vi "Calculate Values Of ScrollBar.vi"(9 "Bounds  Of Picture":T1, 10 "Display Data":T2[](array[typedef]), 11 "Actual Data":T2[](array[typedef])) -> (2 "Total":u32, 3 "index of element":i32, 4 "Max.Scale":i32)   [LabVIEW 2014, in "SmartPalette.lvlib"]
uses:
  SmartPalette.lvlib
  Controls/Palette Data.ctl
  <vilib>/picture/picture.llb/imagedata.ctl
  <vilib>/Utility/miscctls.llb/LVBoundsTypeDef.ctl
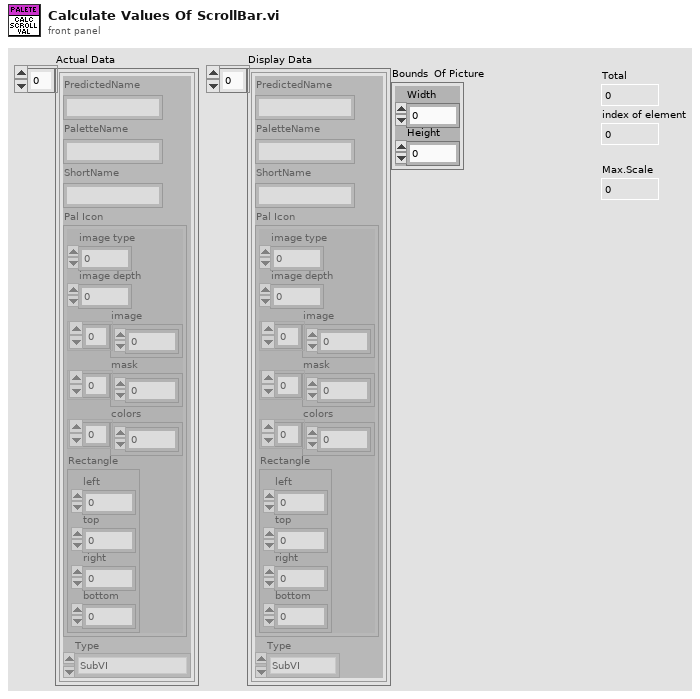
[diagram p1: front panel]
types:
  T1 = typedef "LVBoundsTypeDef.ctl" = cluster{"Width":u32, "Height":u32}
  T2 = typedef "SmartPalette.lvlib/Palette Data.ctl" = cluster{"PredictedName":string, "PaletteName":string, "ShortName":string, "Pal Icon":T3, "Type":enum16{"SubVI", "VI Templtate", "Function"}}
  T3 = typedef "imagedata.ctl" = cluster{"image type":i32, "image depth":i32, "image":u8[], "mask":u8[], "colors":u32[], "Rectangle":cluster{"left":i16, "top":i16, "right":i16, "bottom":i16}}
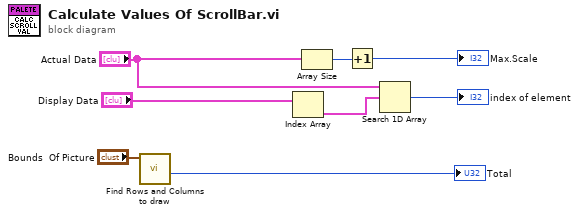
[diagram p0: block diagram]
diagram:
  n1 = call "Find Rows and Columns to draw.vi"("Bounds  Of Picture"="Bounds  Of Picture") -> ("Total"=→"Total":u32)  [unwired: 8 in, 2 out]
  n2 = Index Array(array="Display Data") -> (element=w6:T2)  [unwired: 1 in]
  n3 = Array Size(array="Actual Data") -> (size(s)=w3:i32)
  n4 = Increment(x=w3) -> (x+1=→"Max.Scale":i32)
  n5 = Search 1D Array(1D array="Actual Data", element=w6) -> (index of element=→"index of element":i32)  [unwired: 1 in]
